vi "Grouped_Proj _newa.vi"() -> ()   [LabVIEW 2017]
uses:
  <instrlib>/Lake Shore 336/Public/Data/Sensor Data (Single Reading).vi
  <vilib>/Utility/file.llb/Write Delimited Spreadsheet (DBL).vi
  <instrlib>/Lake Shore 336/Lake Shore 336.lvlib
panel:
  in  "Temp tolerance":dbl
  in  "Temp end":dbl
  in  "step":dbl
  in  "Temp start":dbl
  in  "stop":bool
  in  "Setpoint (0.00000)":dbl format="%.5f"
  in  "Range (0:Off)":u16(ring) items=["Off", "Low (On)", "Medium", "High"]
  in  "Manual Output (0.00 %)":dbl format="%.2f"
  in  "Rate (D) (0.0 %)":dbl format="%.1f"
  in  "Reset (I) (20.0)":dbl=20.0 format="%.1f"
  in  "Gain (P) (50.0)":dbl=50.0 format="%.1f"
  in  "Max Current (0:User Specified)":u16(ring) items=["User Specified", "0.707 A", "1.0 A", "1.141 A", "2.0 A"]
  in  "Mode (0:Off)":u16(ring) items=["Off", "Closed Loop PID", "Zone", "Open Loop"]
  in  "Input (0:None)":u16(ring) items=["None", "A", "B", "C", "D"]
  in  "Output's Control Loop (1:1)":u16(ring)=1 items=["1"=1, "2"=2]
  out "Measured Temperature":dbl format="%.4g"
  in  "Temperature controller address":refnum<visa-resource-name>
  in  "file to save data (dialog if empty)":path
  in  "Resistance Range Lower Limit (2 Ohm)":dbl=2.0 format="%#_6p"
  in  "Resistance Range Upper Limit (2E+8 Ohm)":dbl=200000000.0 format="%#_6p"
  in  "Resistance NPLC (0.1)":dbl=0.1
  in  "Resistance Range (2 Ohm)":dbl=2.0
  in  "Resistance Auto Range (T: Enable)":bool=TRUE
  out "Measured Resistance (Ohms)":dbl format="%#_6p"
  in  "Source Meter address":refnum<visa-resource-name>="GPIB1::29::INSTR"
  in  "Error In":errorcluster
  # "Resistance vs Temperature Measurement"
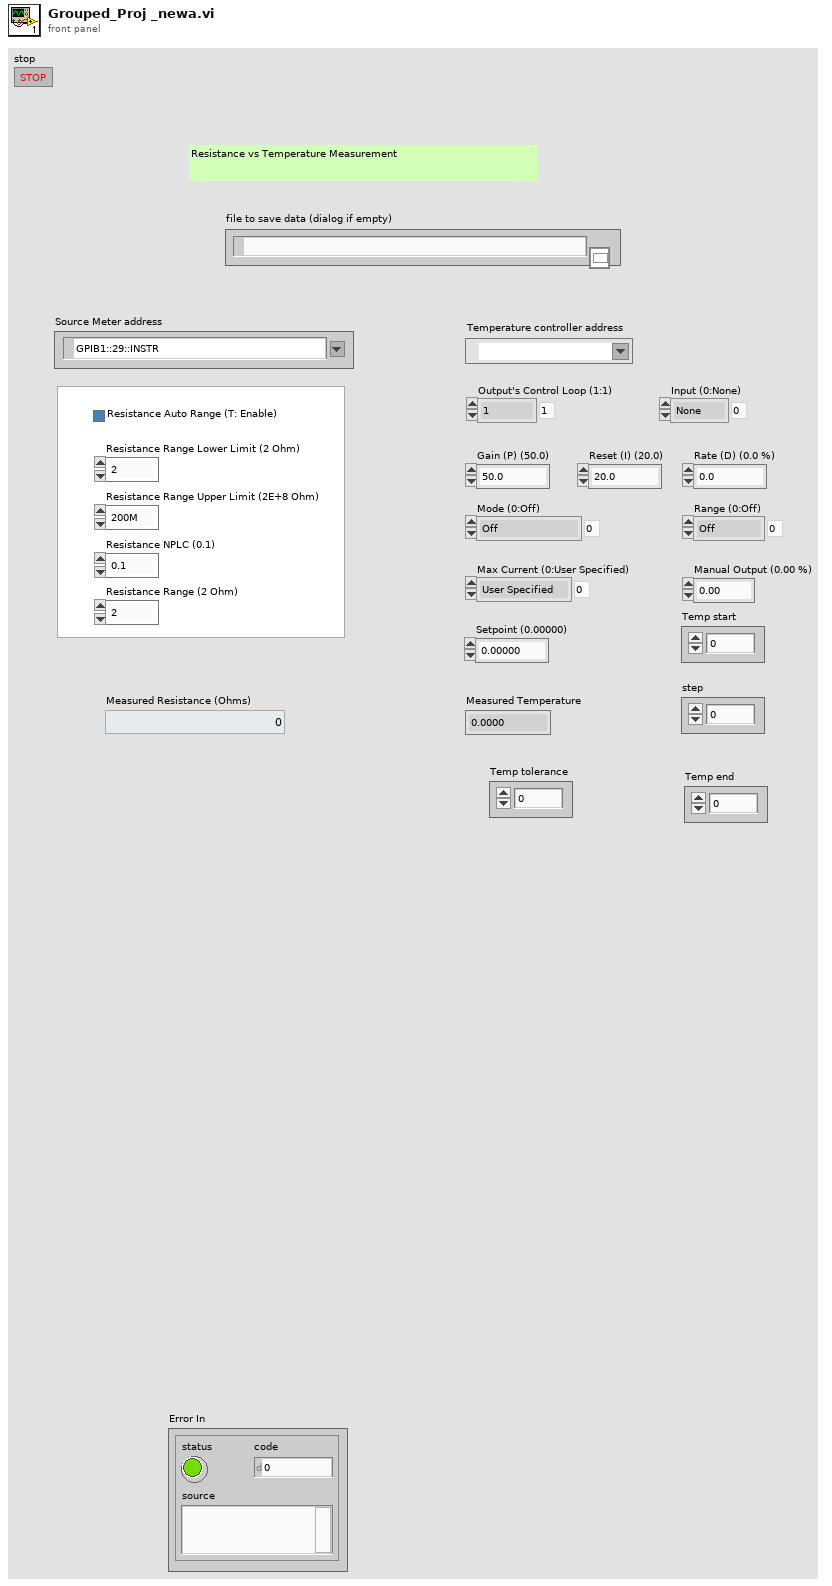
[diagram p1: front panel]
types:
  T1 = cluster{"Baud Rate":u32, "Parity":u16, "Data Bits":u16, "Stop Bits":u16, "Flow Control":u16}
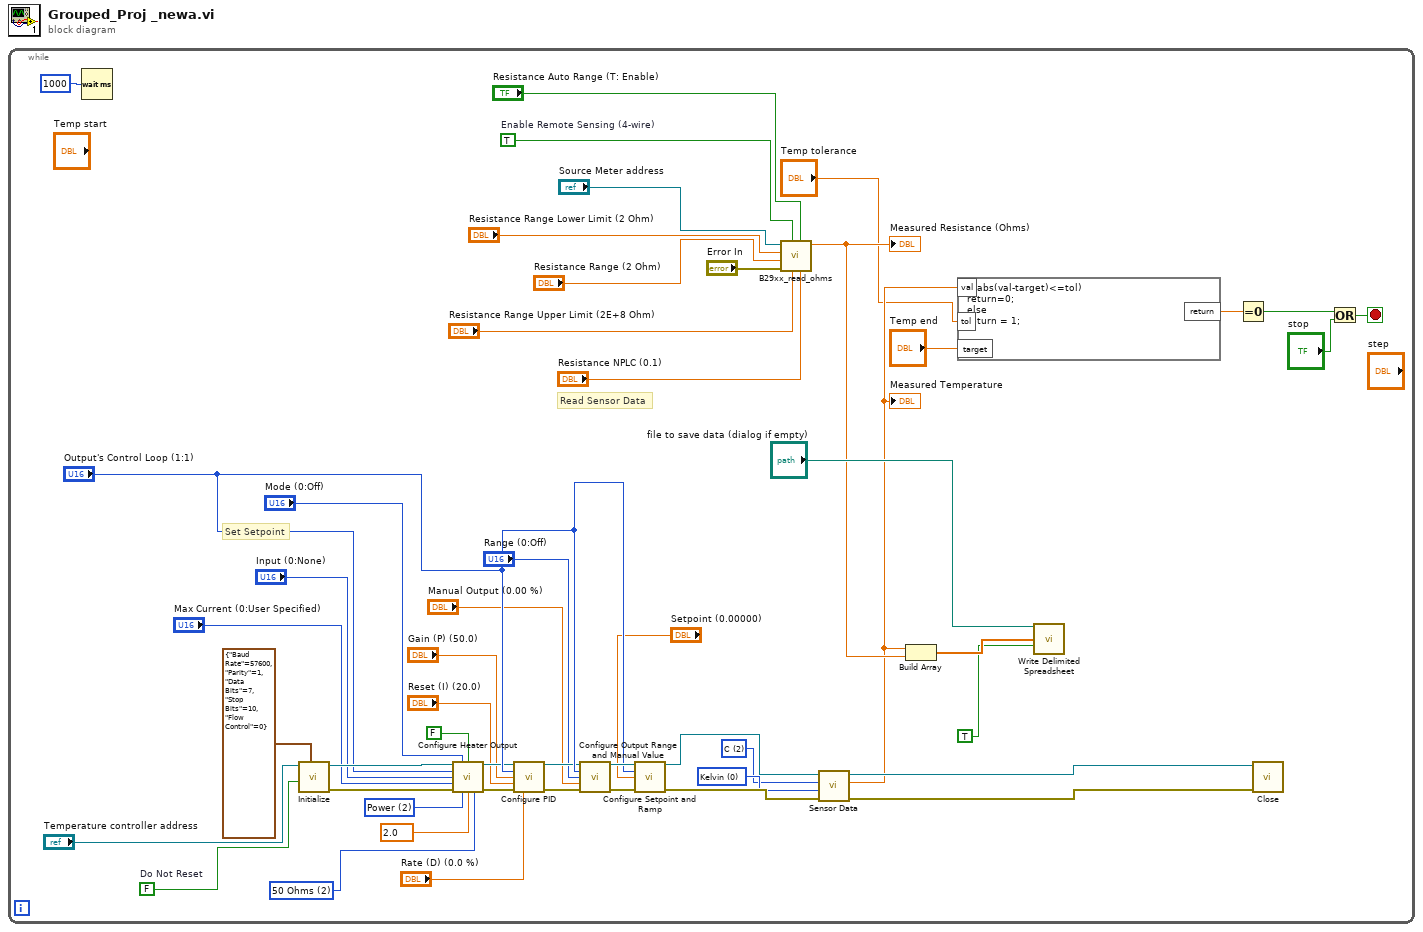
[diagram p0: block diagram]
diagram:
  n1 = while {
    stop <- w6 stop-if-true
    w9 = u16 2 items=["A", "B", "C", "D"] ("Input (0:A)")
    w17 = u16 2 items=["50 Ohms"=2, "25 Ohms"=1] ("Heater Resistance (default to 50Ohms)")
    w30 = u16 0 items=["Kelvin", "Celsius", "Sensor Units"] ("Data Source (0:Kelvin)")
    w19 = u16 2 items=["Current"=1, "Power"=2] ("Heater Out Display (1:Current)")
    w34 = FALSE  # Do Not Reset
    w49 = TRUE  # Enable Remote Sensing (4-wire)
    # "Set Setpoint"
    # "Read Sensor Data"
    n2 = Wait (ms)(milliseconds to wait=u32 1000) -> ()  [unwired: 1 out]
    n3 = call <instrlib>:"Initialize.vi"("Serial Configuration"=T1 {"Baud Rate"=57600, "Parity"=1, "Data Bits"=7, "Stop Bits"=10, "Flow Control"=0}, "Reset (True)"=w34, "VISA resource name"="Temperature controller address") -> ("error out"=w38:errorcluster, "VISA resource name out"=w39:refnum<visa-resource-name>)  [unwired: 7 in]
    n4 = call <instrlib>:"Configure Heater Output.vi"("VISA resource name"=w39, "Mode (0:Off)"="Mode (0:Off)", "Power Up Enable (F: Off)"=FALSE, "Heater Output (1:1)"="Output's Control Loop (1:1)", "Input (0:None)"="Input (0:None)", "Max Current (0:User Specified)"="Max Current (0:User Specified)", "error in (no error)"=w38, "Heater Out Display (1:Current)"=w19, "Max User Current (2.000)"=2.0, "Heater Resistance (1:25 Ohms)"=w17) -> ("VISA resource name out"=w25:refnum<visa-resource-name>, "error out"=w26:errorcluster)  [unwired: 4 in]
    n5 = call <instrlib>:"Configure PID.vi"("VISA resource name"=w25, "Output's Control Loop (1:1)"="Output's Control Loop (1:1)", "Gain (P) (50.0)"="Gain (P) (50.0)", "Reset (I) (20.0)"="Reset (I) (20.0)", "error in (no error)"=w26, "Rate (D) (0.0 %)"="Rate (D) (0.0 %)") -> ("VISA resource name out"=w24:refnum<visa-resource-name>, "error out"=w23:errorcluster)  [unwired: 8 in]
    n6 = call <instrlib>:"Configure Output Range and Manual Value.vi"("VISA resource name"=w24, "Output (1:1)"="Output's Control Loop (1:1)", "Range (0:Off)"="Range (0:Off)", "Manual Output (0.00 %)"="Manual Output (0.00 %)", "error in (no error)"=w23) -> ("VISA resource name out"=w36:refnum<visa-resource-name>, "error out"=w35:errorcluster)  [unwired: 9 in]
    n7 = call <instrlib>:"Configure Setpoint and Ramp.vi"("VISA resource name"=w36, "Output's Control Loop (1:1)"="Output's Control Loop (1:1)", "Setpoint (0.00000)"="Setpoint (0.00000)", "error in (no error)"=w35) -> ("VISA resource name out"=w32:refnum<visa-resource-name>, "error out"=w31:errorcluster)  [unwired: 10 in]
    n8 = call "B29xx_read_ohms.vi"("Resistance NPLC (0.1)"="Resistance NPLC (0.1)", "Resistance Auto Range (T: Enable)"="Resistance Auto Range (T: Enable)", "Resistance Range Upper Limit (2E+8 Ohm)"="Resistance Range Upper Limit (2E+8 Ohm)", "Enable Remote Sensing (4-wire)"=w49, "error in (no error)"="Error In", "Resistance Range (2 Ohm)"="Resistance Range (2 Ohm)", "Resistance Range Lower Limit (2 Ohm)"="Resistance Range Lower Limit (2 Ohm)", "VISA Refnum in"="Source Meter address") -> ("Measurement Result"=w40:dbl)  [unwired: 2 in, 1 out]
    "Measured Resistance (Ohms)" <- w40
    n9 = call-poly <instrlib>:"Sensor Data.vi"("error in (no error)"=w31, "Data Source (0:Kelvin)"=w30, "Input (0:A)"=w9, "VISA resource name"=w32) -> ("error out"=w28:errorcluster, "Sensor Data"=w3:dbl, "VISA resource name out"=w29:refnum<visa-resource-name>)  [unwired: 5 in]
    "Measured Temperature" <- w3
    n10 = Build Array(w3, w40) -> (w42:dbl[])
    n11 = formula code="if(abs(val-target)<=tol)\nreturn=0;\nelse \nreturn = 1;"("val"=w3, "tol"="Temp tolerance", "target"="Temp end") -> ("return"=w4:dbl)
    n12 = call-poly <vilib>:"Write Delimited Spreadsheet.vi"("file path (dialog if empty)"="file to save data (dialog if empty)", "1D data"=w42, "append to file? (new file:F)"=TRUE) -> ()  [unwired: 11 in, 2 out]
    n13 = Equal To 0?(x=w4) -> (x = 0?=w5:bool)
    n14 = call <instrlib>:"Close.vi"("error in (no error)"=w28, "VISA resource name"=w29) -> ()  [unwired: 9 in, 1 out]
    n15 = Or(x=w5, y="stop") -> (x .or. y?=w6:bool)
  }
